vi "CLSUIP_FindImplementation.vi"(3 "error in":errorcluster, 4 "Method Name":string, 5 "Class in":refnum<vi>) -> (0 "error out":errorcluster, 1 "VI":refnum<vi>, 2 "Class out":refnum<vi>)   [LabVIEW 2021, in "ChooseImplementation.lvlib"]
uses:
  <resource>/Framework/Providers/LVClassLibrary/ChooseImplementation/ChooseImplementation.lvlib
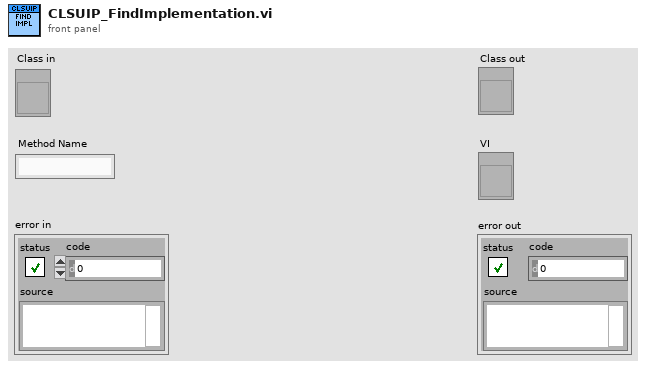
[diagram p1: front panel]
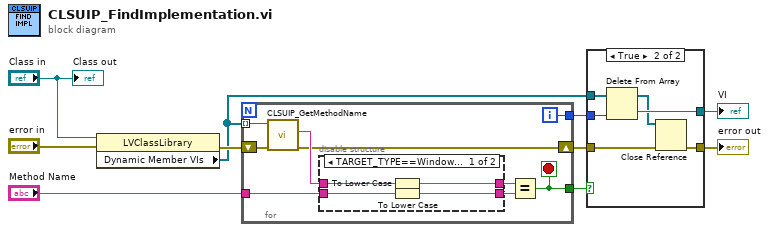
[diagram p0: block diagram]
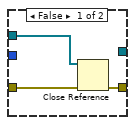
[diagram p2: hidden frame]
diagram:
  n1 = property class="LVClassLibrary"(reference="Class in", error in="error in") -> (error out=w8:errorcluster, "Dynamic Member VIs"=w3:refnum<vi>[])  [unwired: 1 out]
  n2 = for {
    shift-right: [w15] -> w4
    shift-left: w8 -> [w18]
    tunnel: w3 -> [w19] mode=indexing
    tunnel: "Method Name" -> [w16]
    tunnel: [w12] -> w5
    tunnel: [w11] -> w6
    i -> [w11]
    stop <- w12 stop-if-true
    n3 = call <resource>:"CLSUIP_GetMethodName.vi"("error in (no error)"=w18, "VI Reference"=w19) -> ("error out"=w15:errorcluster, "Method Name"=w17:string)  [unwired: 7 in, 1 out]
    n4 = disable-structure shown="TARGET_TYPE==Windows" {
      disable-tunnel: w17 -> [w23 w25]
      disable-tunnel: w16 -> [w22 w24]
      disable-tunnel: [w21 w25] -> w14
      disable-tunnel: [w20 w24] -> w13
      frame condition #0 (active) {
        n5 = To Lower Case(string=w23) -> (all lower case string=w21:string)
        n6 = To Lower Case(string=w22) -> (all lower case string=w20:string)
      }
      frame condition #1 {
      }
    }
    n7 = Equal?(x=w14, y=w13) -> (x = y?=w12:bool)
  }
  n8 = case shown="True" w5 {
    tunnel: w6 -> [_ w32]
    tunnel: w4 -> [w28 w31]
    tunnel: w3 -> [w27 w34]
    tunnel: [w26 w30] -> w2
    tunnel: [_ w33] -> w1
    frame False {
      n9 = Close Reference(reference=w27, error in (no error)=w28) -> (error out=w26:errorcluster)
    }
    frame True {
      n10 = Delete From Array(array=w34, index=w32) -> (deleted portion=w33:refnum<vi>, array with subset deleted=w29:refnum<vi>[])  [unwired: 1 in]
      n11 = Close Reference(reference=w29, error in (no error)=w31) -> (error out=w30:errorcluster)
    }
  }
  "VI" <- w1
  "error out" <- w2
  "Class out" <- "Class in"
